vi "FormulaNodeUse_Sine_WaveGraph.vi"() -> ()   [LabVIEW 2017]
panel:
  out "Array":dbl[](array[numeric])
  out "Waveform Graph":cluster{dbl, dbl, dbl[]}(graph)
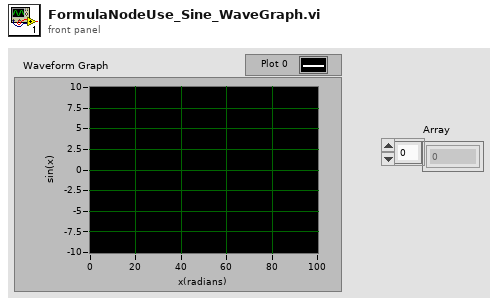
[diagram p1: front panel]
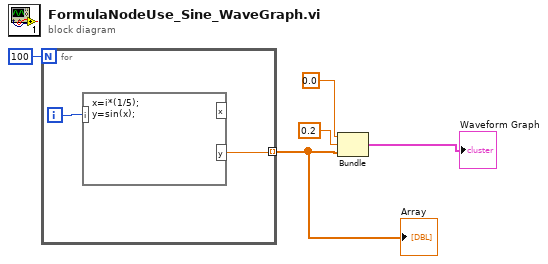
[diagram p0: block diagram]
diagram:
  n1 = for {
    N: 100 -> [_]
    tunnel: [w6] -> w1 mode=indexing
    i -> [w7]
    n2 = formula code="x=i*(1/5);\ny=sin(x);"("i"=w7) -> ("y"=w6:dbl)  [unwired: 1 out]
  }
  "Array" <- w1
  n3 = Bundle(0.0, 0.2, w1) -> (→"Waveform Graph":cluster{dbl, dbl, dbl[]})  [unwired: 1 in]
